vi "Configure Output Off Behavior.vi"(8 "error in (no error)":errorcluster, 9 "Function (0: Volts)":u16(ring) items=["Volts", "Current"], 10 "Output Off Behavior (0: Normal)":u16(ring) items=["Normal", "High Impedance", "Zero", "Guard"], 11 "VISA resource name":refnum<visa-resource-name>) -> (0 "error out":errorcluster, 3 "VISA resource name out":refnum<visa-resource-name>)   [LabVIEW 2022 SP3, in "Keithley 2450.lvlib"]
doc: "Configures the instrument's behavior when the output is disabled."
uses:
  Keithley 2450.lvlib
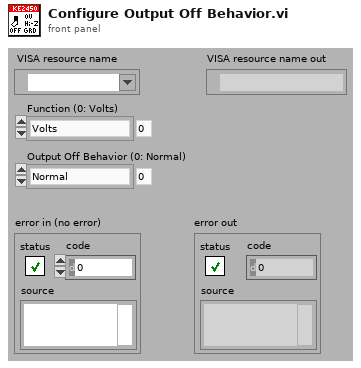
[diagram p1: front panel]
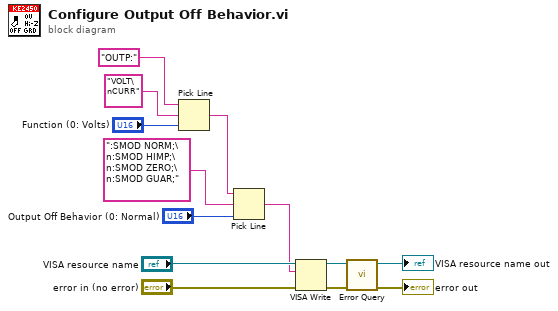
[diagram p0: block diagram]
diagram:
  n1 = Pick Line(string ("")="OUTP:", multi-line string="VOLT\nCURR", line index="Function (0: Volts)") -> (output string=w1:string)
  n2 = Pick Line(string ("")=w1, multi-line string=":SMOD NORM;\n:SMOD HIMP;\n:SMOD ZERO;\n:SMOD GUAR;", line index="Output Off Behavior (0: Normal)") -> (output string=w9:string)
  n3 = VISA Write(VISA resource name="VISA resource name", write buffer=w9, error in (no error)="error in (no error)") -> (VISA resource name out=w8:refnum<visa-resource-name>, error out=w5:errorcluster)  [unwired: 1 out]
  n4 = call "Error Query.vi"("error in (no error)"=w5, "VISA resource name"=w8) -> ("error out"=→"error out":errorcluster, "VISA resource name out"=→"VISA resource name out":refnum<visa-resource-name>)  [unwired: 8 out]
